vi "send-command.vi"(8 "parameters":string="{}", 9 "command":string="get wnum", 11 "target":cluster{"port":i32, "host":string}={"port"=8250, "host"="127.0.0.1"}) -> (0 "error out":errorcluster, 3 "output":string)   [LabVIEW 2014]
uses:
  <vilib>/httpClient/POSTBuffer.vi
  <vilib>/httpClient/LabVIEWHTTPClient.lvlib
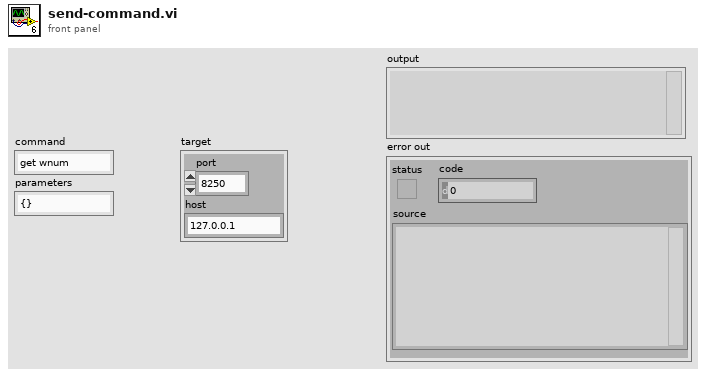
[diagram p1: front panel]
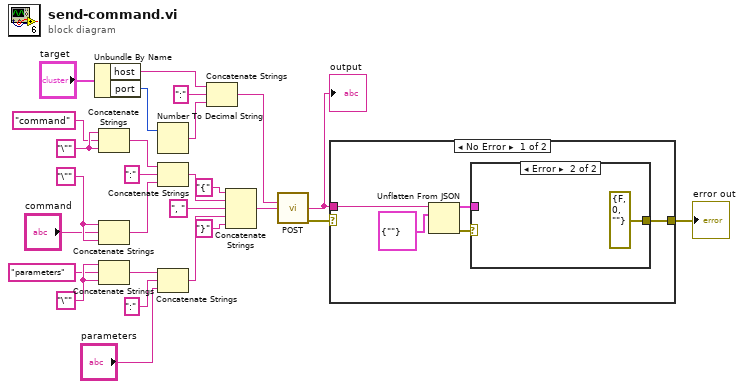
[diagram p0: block diagram]
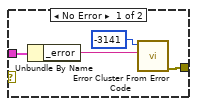
[diagram p2: hidden frame]
diagram:
  w13 = "\"" ("string")
  w19 = "\"" ("string")
  w21 = "\"" ("string")
  n1 = Unbundle By Name("target") -> ("host"=w5:string, "port"=w4:i32)
  n2 = Concatenate Strings(w21, "command" ("string"), w21) -> (w17:string)
  n3 = Concatenate Strings(w13, "command", w13) -> (w11:string)
  n4 = Concatenate Strings(w19, "parameters" ("string"), w19) -> (w14:string)
  n5 = Number To Decimal String(number=w4) -> (decimal integer string=w26:string)  [unwired: 1 in]
  n6 = Concatenate Strings(w17, ":" ("string"), w11) -> (w10:string)
  n7 = Concatenate Strings(w14, ":" ("string"), "parameters") -> (w9:string)
  n8 = Concatenate Strings(w5, ":" ("string"), w26) -> (w25:string)
  n9 = Concatenate Strings("{" ("string"), w10, ", " ("string"), w9, "}" ("string")) -> (w8:string)
  n10 = call-poly <vilib>:"POST.vi"("url"=w25, "buffer"=w8) -> ("body"=w3:string, "error out"=w2:errorcluster)  [unwired: 10 in, 2 out]
  "output" <- w3
  n11 = case shown="No Error" w2 {
    selector: w2 -> [_ w38]
    tunnel: w3 -> [w31 _]
    tunnel: [w28 w38] -> w1
    frame No Error {
      n12 = Unflatten From JSON(JSON string=w31, type and defaults=cluster{"_error":string} {"_error"=""}) -> (value=w29:cluster{"_error":string}, error out=w30:errorcluster)  [unwired: 5 in]
      n13 = case shown="Error" w30 {
        tunnel: w29 -> [w36 _]
        tunnel: [w33 errorcluster {"status"=FALSE, "code"=0, "source"=""} ("error constant")] -> w28
        frame No Error {
          n14 = Unbundle By Name(w36) -> ("_error"=w35:string)
          n15 = call <vilib>:"Error Cluster From Error Code.vi"("error message (\"\")"=w35, "error code (0)"=-3141 ("code")) -> ("error out"=w33:errorcluster)  [unwired: 7 in]
        }
        frame Error {
        }
      }
    }
    frame Error {
    }
  }
  "error out" <- w1
